vi "Validate Range.vi"(8 "error in (no error)":errorcluster, 10 "Range":T1, 11 "DAQ Digital Code Scan in":refnum<class "DAQ Digital Code Scan.lvclass">) -> (0 "error out":errorcluster, 2 "Validated Range":T1, 3 "DAQ Digital Code Scan out":refnum<class "DAQ Digital Code Scan.lvclass">)   [LabVIEW 2012, in "DAQ Digital Code Scan.lvclass"]
doc: "Coerce the range to be within this Scanner's physical limits."
uses:
  DAQ Digital Code Scan.lvclass
  Scanner/Range.ctl
  LabVIEW-programs/Scanners/Scanner/Scanner.lvclass
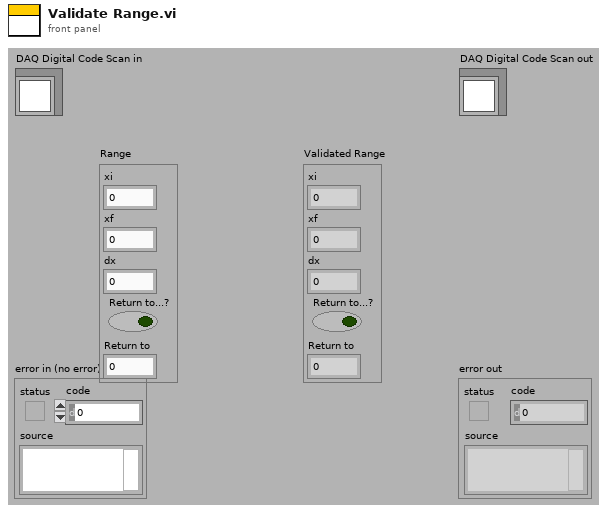
[diagram p1: front panel]
types:
  T1 = typedef "Scanner.lvclass/Range.ctl" = cluster{"xi":dbl, "xf":dbl, "dx":dbl, "Return to...?":bool, "Return to":dbl}
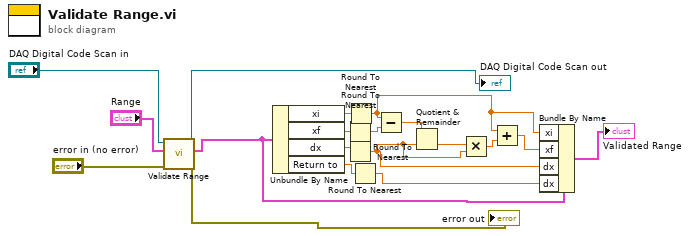
[diagram p0: block diagram]
diagram:
  n1 = call-parent "Validate Range.vi"("error in (no error)"="error in (no error)", "Range"="Range", "Scanner in"="DAQ Digital Code Scan in") -> ("error out"=→"error out":errorcluster, "Validated Range"=w7:T1, "Scanner out"=→"DAQ Digital Code Scan out":refnum<class "DAQ Digital Code Scan.lvclass">)  [unwired: 6 in]
  n2 = Unbundle By Name(w7) -> ("xi"=w14:dbl, "xf"=w13:dbl, "dx"=w12:dbl, "Return to"=w6:dbl)
  n3 = Round To Nearest(number=w13) -> (nearest integer value=w11:dbl)
  n4 = Round To Nearest(number=w12) -> (nearest integer value=w4:dbl)
  n5 = Round To Nearest(number=w14) -> (nearest integer value=w2:dbl)
  n6 = Round To Nearest(number=w6) -> (nearest integer value=w5:dbl)
  n7 = Subtract(x=w2, y=w11) -> (x-y=w10:dbl)
  n8 = Quotient & Remainder(x=w10, y=w4) -> (floor(x/y)=w9:dbl)  [unwired: 1 out]
  n9 = Multiply(x=w9, y=w4) -> (x*y=w8:dbl)
  n10 = Add(x=w2, y=w8) -> (x+y=w3:dbl)
  n11 = Bundle By Name(cluster=w7, "xi"=w2, "xf"=w3, "dx"=w4, "dx"=w5) -> (→"Validated Range":T1)
